vi "Start Trigger.vi"(8 "error in":errorcluster, 11 "4300 in":refnum<class "4300.lvclass">) -> (0 "error out":errorcluster, 3 "4300 out":refnum<class "4300.lvclass">)   [LabVIEW 2019, in "4300.lvlib" / "4300.lvclass"]
uses:
  Library/4300.lvclass
  C:/Users/Public/Documents/Development/builds/Instruments/AnalogInput.lvlibp/Library/AnalogInput.lvclass
  builds/Instruments/AnalogInput.lvlibp/Accessors/Triggering/Read Enable Digital Trigger.vi
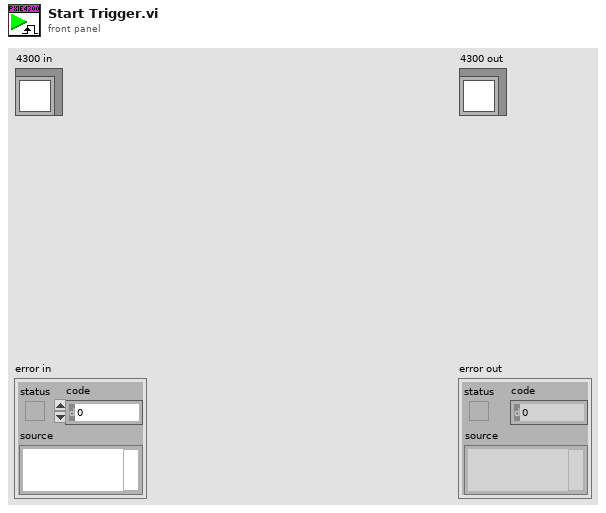
[diagram p1: front panel]
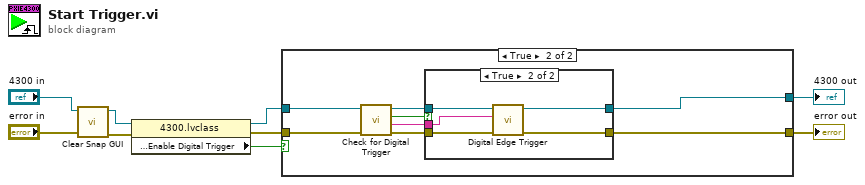
[diagram p0: block diagram]
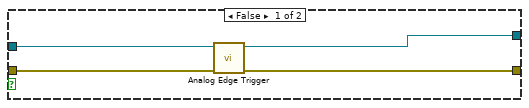
[diagram p2: hidden frame]
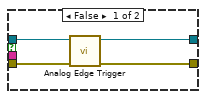
[diagram p3: hidden frame]
diagram:
  n1 = call "Clear Snap GUI.vi"("error in (no error)"="error in", "4300 in"="4300 in") -> ("error out"=w3:errorcluster, "4300 out"=w2:refnum<class "4300.lvclass">)  [unwired: 8 in]
  n2 = property class="4300.lvclass"(reference=w2, error in=w3) -> (reference out=w7:refnum<class "4300.lvclass">, error out=w5:errorcluster, "Accessors:Config:Enable Digital Trigger"=w6:bool)
  n3 = case shown="True" w6 {
    tunnel: [w10 w21] -> w9
    tunnel: [w11 w20] -> w8
    tunnel: w7 -> [w12 w19]
    tunnel: w5 -> [w13 w18]
    frame False {
      n4 = call "Analog Edge Trigger.vi"("error in (no error)"=w13, "4300 in"=w12) -> ("error out"=w10:errorcluster, "4300 out"=w11:refnum<class "4300.lvclass">)  [unwired: 8 in]
    }
    frame True {
      n5 = call "Check for Digital Trigger.vi"("error in (no error)"=w18, "4300 in"=w19) -> ("error out"=w16:errorcluster, "TriggerSource"=w14:string, "IsDigital"=w15:bool, "4300 out"=w17:refnum<class "4300.lvclass">)  [unwired: 6 in]
      n6 = case shown="True" w15 {
        tunnel: [w22 w26] -> w21
        tunnel: [w23 w27] -> w20
        tunnel: w17 -> [w25 w30]
        tunnel: w16 -> [w24 w29]
        tunnel: w14 -> [_ w28]
        frame False {
          n7 = call "Analog Edge Trigger.vi"("error in (no error)"=w24, "4300 in"=w25) -> ("error out"=w22:errorcluster, "4300 out"=w23:refnum<class "4300.lvclass">)  [unwired: 8 in]
        }
        frame True {
          n8 = call "Digital Edge Trigger.vi"("error in"=w29, "Source"=w28, "4300 in"=w30) -> ("error out"=w26:errorcluster, "4300 out"=w27:refnum<class "4300.lvclass">)  [unwired: 7 in]
        }
      }
    }
  }
  "error out" <- w9
  "4300 out" <- w8
